vi "MFIA Filter Response Calculation.vi"(10 "Filter order":i32 min=0 max=8 step=1, 11 "Bandwidth":dbl[unit]=1.0 min=1.0) -> (2 "Settling times":T1 {"T_s 50%" format="%#_6p"; "T_s 1-1/e" format="%#_6p"; "T_s 90%" format="%#_6p"; "T_s 95%" format="%#_6p"; "T_s 99%" format="%#_6p"}, 3 "TC":dbl[unit] format="%#_6p")   [LabVIEW 2019]
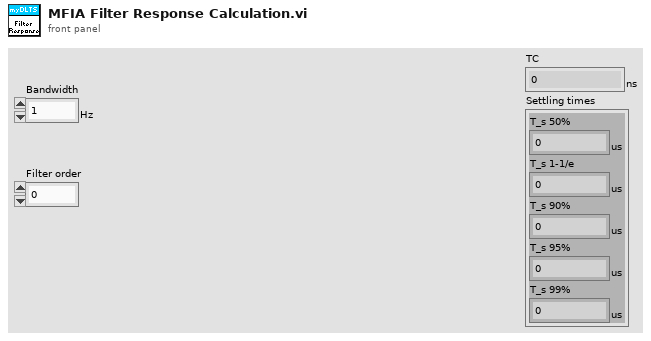
[diagram p1: front panel]
types:
  T1 = cluster{"T_s 50%":dbl[unit], "T_s 1-1/e":dbl[unit], "T_s 90%":dbl[unit], "T_s 95%":dbl[unit], "T_s 99%":dbl[unit]}
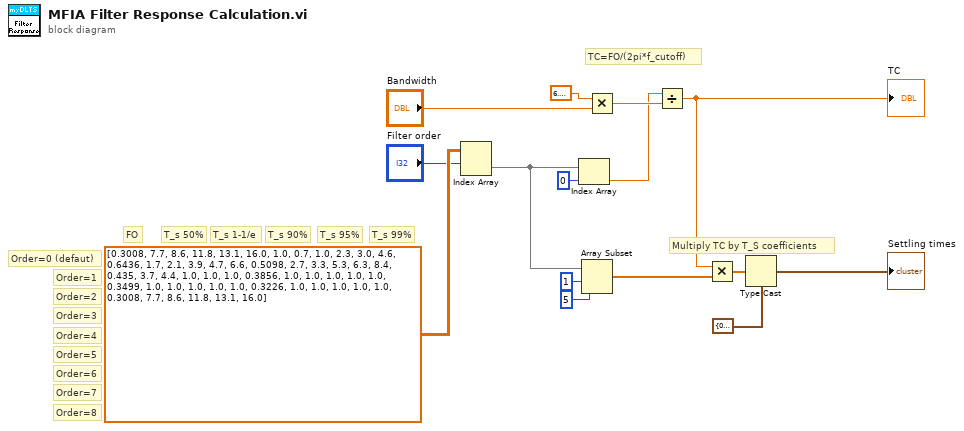
[diagram p0: block diagram]
diagram:
  # "TC=FO/(2pi*f_cutoff)"
  # "Multiply TC by T_S coefficients"
  # "Order=8"
  # "Order=7"
  # "Order=6"
  # "Order=5"
  # "Order=4"
  # "Order=3"
  # "Order=2"
  # "Order=1"
  # "Order=0 (defaut)"
  # "T_s 1-1/e"
  # "T_s 99%"
  # "T_s 95%"
  # "T_s 90%"
  # "T_s 50%"
  # "FO"
  n1 = Index Array(array=dbl[][] [[0.3008, 7.7, 8.6, 11.8, 13.1, 16.0], [1.0, 0.7, 1.0, 2.3, 3.0, 4.6], [0.6436, 1.7, 2.1, 3.9, 4.7, 6.6], [0.5098, 2.7, 3.3, 5.3, 6.3, 8.4], [0.435, 3.7, 4.4, 1.0, 1.0, 1.0], [0.3856, 1.0, 1.0, 1.0, 1.0, 1.0], [0.3499, 1.0, 1.0, 1.0, 1.0, 1.0], [0.3226, 1.0, 1.0, 1.0, 1.0, 1.0], [0.3008, 7.7, 8.6, 11.8, 13.1, 16.0]], index (row)="Filter order") -> (element=w8:dbl[])  [unwired: 1 in]
  n2 = Index Array(array=w8, index=0) -> (element=w9:dbl)
  n3 = Array Subset(array=w8, index=1, length=5) -> (w5:dbl[])
  n4 = Multiply(x=6.283185307179586, y="Bandwidth") -> (x*y=w14:dbl[unit])
  n5 = Divide(x=w9, y=w14) -> (x/y=w4:dbl[unit])
  "TC" <- w4
  n6 = Multiply(x=w4, y=w5) -> (x*y=w3:dbl[unit][])
  n7 = Type Cast(type=T1 {"T_s 50%"=0.0, "T_s 1-1/e"=0.0, "T_s 90%"=0.0, "T_s 95%"=0.0, "T_s 99%"=0.0}, x=w3) -> (*(type *) &x=→"Settling times":T1)
